vi "PDF Standard Kopf Gas Flasche.vi"(8 "Verdünnungsgas":T1 items=["N2", "O2"], 9 "Ablaufdatum":timestamp, 10 "Genauigkeit in":dbl, 11 "Gaschflasche Auswahl Cluster":T3) -> (0 "Konzentration":string, 1 "Ablaufdatum":string, 2 "Genauigkeit":string, 3 "Chargennummer":string, 4 "Gasauswahl":string, 5 "Gasname für die Auswahl":string, 6 "Trägergas":T2="N2")   [LabVIEW 2020, in "PDF Interface.lvlib"]
uses:
  PDF Interface.lvlib
  PDF Protokoll Standard Kopf Gasflasche Auswahl.ctl
  Seiten/System Einstellungen V2/Traegergas.ctl
  Seiten/System Einstellungen V2/Gasflasche.ctl
  Seiten/System Einstellungen V2/Aktion FGV Gasbottledefinition.ctl
  Seiten/System Einstellungen V2/System Einstellungen V2.lvlib
  Linearisierung V2/SpanEinstellungen/SpanEinstellungen.lvlib
  Linearisierung V2/Gasteiler/Gasteiler.lvlib
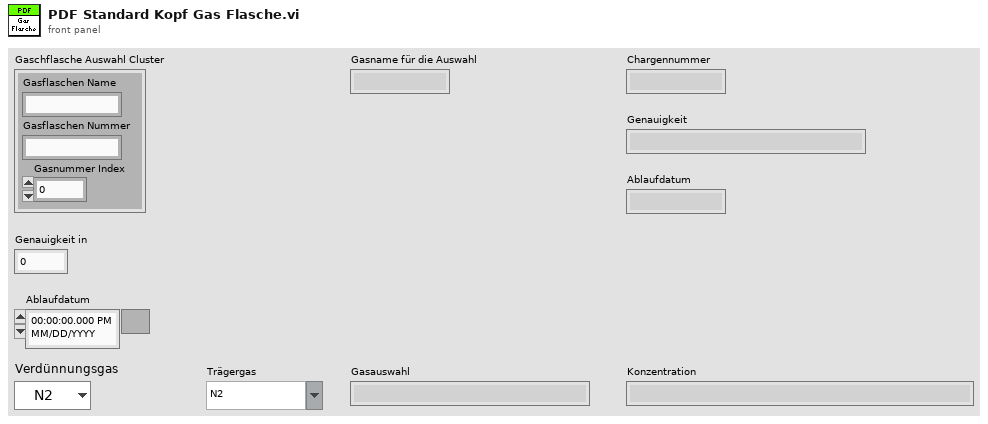
[diagram p1: front panel]
types:
  T1 = typedef "Linearisierung v2.lvlib/Gasteiler.lvlib/Prüfgas in.ctl" = u16
  T2 = typedef "System Einstellungen V2.lvlib/Traegergas.ctl" = string
  T3 = typedef "PDF Interface.lvlib/PDF Protokoll Standard Kopf Gasflasche Auswahl.ctl" = cluster{"Gasflaschen Name":string, "Gasflaschen Nummer":string, "Gasnummer Index":i32}
  T4 = typedef "System Einstellungen V2.lvlib/Aktion FGV Gasbottledefinition.ctl" = enum16{"lesen", "schreiben", "löschen", "laden", "speichern", "exportieren", "importieren"}
  T5 = typedef "System Einstellungen V2.lvlib/Gasflasche.ctl" = cluster{"Gasname für die Auswahl":string, "Chargennummer":string, "Ablaufdatum":timestamp}
  T6 = typedef "System Einstellungen V2.lvlib/Gasflasche gesamt.ctl" = cluster{"Gasflasche":T5, "Trägergas":T2, "Komponenten":T7[]}
  T7 = typedef "System Einstellungen V2.lvlib/Gasflaschenkomponente.ctl" = cluster{"Gasauswahl":string, "Konzentration IST":dbl, "Einheit":string, "Genauigkeit":dbl}
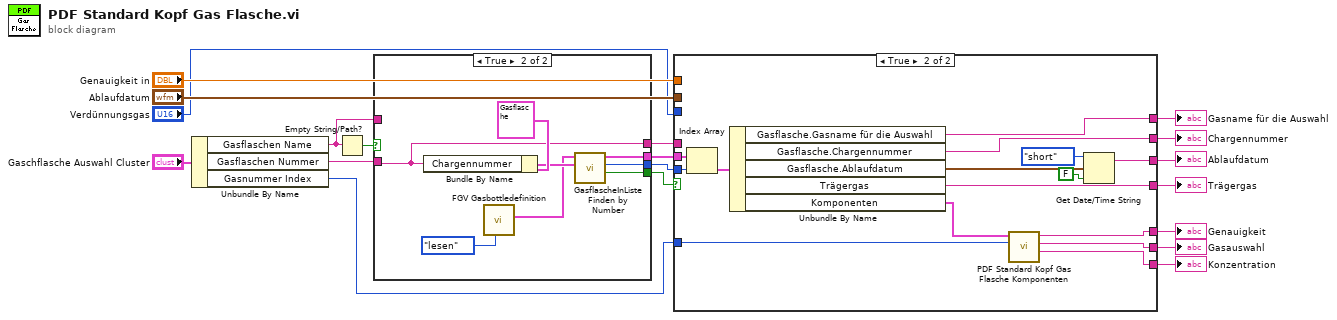
[diagram p0: block diagram]
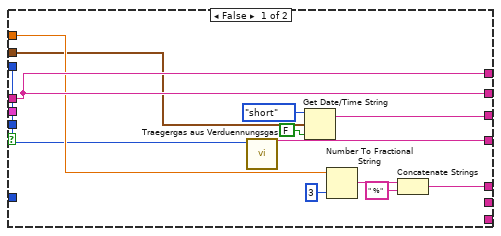
[diagram p2: hidden frame]
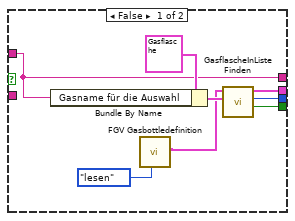
[diagram p3: hidden frame]
diagram:
  n1 = Unbundle By Name("Gaschflasche Auswahl Cluster") -> ("Gasflaschen Name"=w16:string, "Gasflaschen Nummer"=w17:string, "Gasnummer Index"=w8:i32)
  n2 = Empty String/Path?(string/path=w16) -> (empty?=w18:bool)
  n3 = case shown="True" w18 {
    tunnel: w17 -> [_ w28]
    tunnel: w16 -> [w20 _]
    tunnel: [w23 w31] -> w15
    tunnel: [w22 w30] -> w13
    tunnel: [w21 w29] -> w12
    tunnel: [w20 w28] -> w14
    frame False {
      n4 = Bundle By Name(cluster=T5 {"Gasname für die Auswahl"="", "Chargennummer"="", "Ablaufdatum"=timestamp(0 s since 1904-01-01)} ("Gasflasche"), "Gasname für die Auswahl"=w20) -> (w26:T5)
      n5 = call "FGV Gasbottledefinition.vi"("Aktion"=Aktion_FGV_Gasbottledefinition."lesen") -> ("Gasflaschen Liste gesamt"=w24:T6[])  [unwired: 8 in, 2 out]
      n6 = call "GasflascheInListeFinden.vi"("Gasflasche"=w26, "GasflaschenListe"=w24) -> ("gefunden"=w21:bool, "Index"=w22:i32, "GasflaschenListe out"=w23:T6[])  [unwired: 7 in]
    }
    frame True {
      n7 = Bundle By Name(cluster=T5 {"Gasname für die Auswahl"="", "Chargennummer"="", "Ablaufdatum"=timestamp(0 s since 1904-01-01)} ("Gasflasche"), "Chargennummer"=w28) -> (w34:T5)
      n8 = call "FGV Gasbottledefinition.vi"("Aktion"=Aktion_FGV_Gasbottledefinition."lesen") -> ("Gasflaschen Liste gesamt"=w32:T6[])  [unwired: 8 in, 2 out]
      n9 = call "GasflascheInListeFinden by Number.vi"("Gasflasche"=w34, "GasflaschenListe"=w32) -> ("gefunden"=w29:bool, "Index"=w30:i32, "GasflaschenListe out"=w31:T6[])  [unwired: 7 in]
    }
  }
  n10 = case shown="True" w12 {
    tunnel: w15 -> [_ w62]
    tunnel: w13 -> [_ w61]
    tunnel: [w42 w59] -> w5
    tunnel: [w47 w58] -> w11
    tunnel: w14 -> [w47 _]
    tunnel: [w47 w57] -> w10
    tunnel: [w36 w56] -> w9
    tunnel: w8 -> [_ w53]
    tunnel: [_ w55] -> w7
    tunnel: [_ w54] -> w4
    tunnel: "Genauigkeit in" -> [w43 _]
    tunnel: [w38 w49] -> w3
    tunnel: "Ablaufdatum" -> [w39 _]
    tunnel: "Verdünnungsgas" -> [w37 _]
    frame False {
      n11 = call "Traegergas aus Verduennungsgas.vi"("Verdünnungsgas"=w37) -> ("Trägergas"=w36:T2)  [unwired: 10 in]
      n12 = Get Date/Time String(date format (0)=enum16{"short", "long", "abbreviated"}."short" ("Datumsformat (0)"), seconds (now)=w39, want seconds? (F)=FALSE ("Angabe von Sekunden? (F)")) -> (date string=w38:string)  [unwired: 1 out]
      n13 = Number To Fractional String(number=w43, precision (6)=i16 3 ("Genauigkeit (6)")) -> (F-format string=w45:string)  [unwired: 2 in]
      n14 = Concatenate Strings(w45, " %" ("String")) -> (w42:string)
    }
    frame True {
      n15 = Index Array(array=w62, index=w61) -> (element=w60:T6)
      n16 = Unbundle By Name(w60) -> ("Gasflasche.Gasname für die Auswahl"=w57:string, "Gasflasche.Chargennummer"=w58:string, "Gasflasche.Ablaufdatum"=w51:timestamp, "Trägergas"=w56:T2, "Komponenten"=w52:T7[])
      n17 = call "PDF Standard Kopf Gas Flasche Komponenten.vi"("Gasnummer Index"=w53, "Komponenten"=w52) -> ("Konzentration IST"=w54:string, "Gasauswahl"=w55:string, "Genauigkeit"=w59:string)  [unwired: 7 in]
      n18 = Get Date/Time String(date format (0)=enum16{"short", "long", "abbreviated"}."short" ("Datumsformat (0)"), seconds (now)=w51, want seconds? (F)=FALSE ("Angabe von Sekunden? (F)")) -> (date string=w49:string)  [unwired: 1 out]
    }
  }
  "Ablaufdatum" <- w3
  "Chargennummer" <- w11
  "Genauigkeit" <- w5
  "Gasname für die Auswahl" <- w10
  "Trägergas" <- w9
  "Konzentration" <- w4
  "Gasauswahl" <- w7
